vi "cmc-Series-Iterated-Loop.vi"() -> ()   [LabVIEW 2010]
uses:
  <vilib>/gmath/NI_Gmath.lvlib
panel:
  in  "Delay Time (s)":dbl=1.0 min=0.0
  out "\"Canned Solution\"":dbl format="%#_18g"
  out "i-th term":dbl format="%#_18g"
  out "Partial Sum":dbl format="%#_18g"
  out "Total Summation":dbl format="%#_18g"
  in  "Number of Iterations\nRequested":u8
  in  "Theta(radians)":dbl
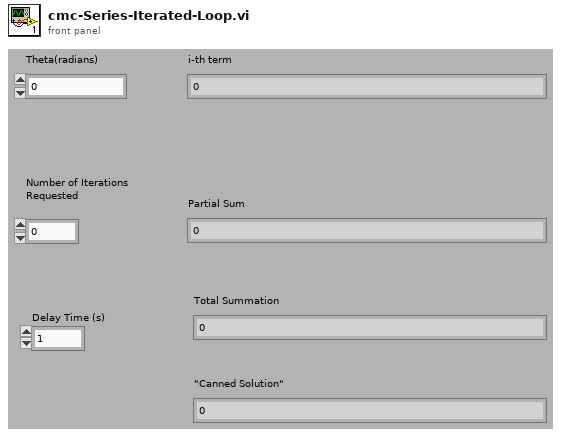
[diagram p1: front panel]
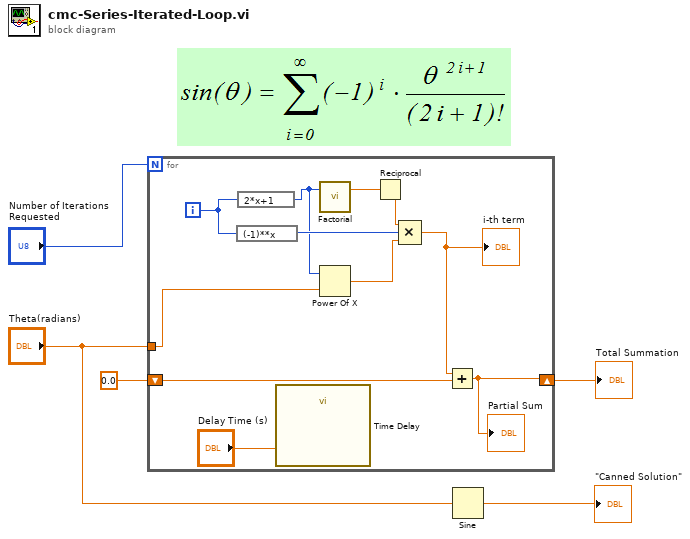
[diagram p0: block diagram]
diagram:
  n1 = for {
    N: "Number of Iterations\nRequested" -> [_]
    tunnel: "Theta(radians)" -> [w9]
    shift-right: [w7] -> w3
    shift-left: 0.0 -> [w12]
    i -> [w15]
    n2 = expression code="(-1)**x"(w15) -> (w14:i32)
    n3 = expression code="2*x+1"(w15) -> (w10:i32)
    n4 = call "Time Delay"("Delay Time (s)"="Delay Time (s)") -> ()  [unwired: 10 in, 1 out]
    n5 = call <vilib>:"Factorial.vi"("n"=w10) -> ("n!"=w11:dbl)  [unwired: 2 in]
    n6 = Power Of X(1:w9, 2:w10) -> (0:w13:dbl)
    n7 = Reciprocal(x=w11) -> (1/x=w16:dbl)
    n8 = Compound Arithmetic op=MULTIPLY(w16, w14, w13) -> (w8:dbl)
    "i-th term" <- w8
    n9 = Add(x=w8, y=w12) -> (x+y=w7:dbl)
    "Partial Sum" <- w7
  }
  "Total Summation" <- w3
  n10 = Sine(x="Theta(radians)") -> (sin(x)=→"\"Canned Solution\"":dbl)
